vi "FRCts20_Backend_SetSglTeamData.vi"(8 "error in (no error)":errorcluster, 11 "Team":T1) -> (0 "error out":errorcluster, 2 "Status?":string)   [LabVIEW 2013, in "FRCts20_Backend_WebMethods.lvlib"]
doc: "The SetSglTeamData function applies a new team description to the data set, or overwrites existing team information with updated values. The function accepts a full team description as input, and provides a <b>Success!</b> or <b>Failed!</b> status return."
uses:
  FRCts20_Backend_WebMethods.lvlib
  FRCts20_Backend_FGVOperation.ctl
  FRCts20_Backend_Engine.lvlib
  FRCts20_Backend_IssueDfn.ctl
  FRCts20_Backend_Controls.lvlib
  FRCts20_Backend_TeamDfn.ctl
  FRCts20_Backend_Team_Info.ctl
  FRCts20_Backend_Note.ctl
  FRCts20_Backend_Note_list.ctl
  FRCts20_Backend_request_info.ctl
  FRCts20_Backend_IssueTeamList.ctl
panel:
  # "The SetSglTeamData function applies a new \nteam description to the data set, or overwrites \nexisting team information with updated values.\nThe function accepts a full team description as\ninput, and provides a Success! or Failed! status\nreturn."
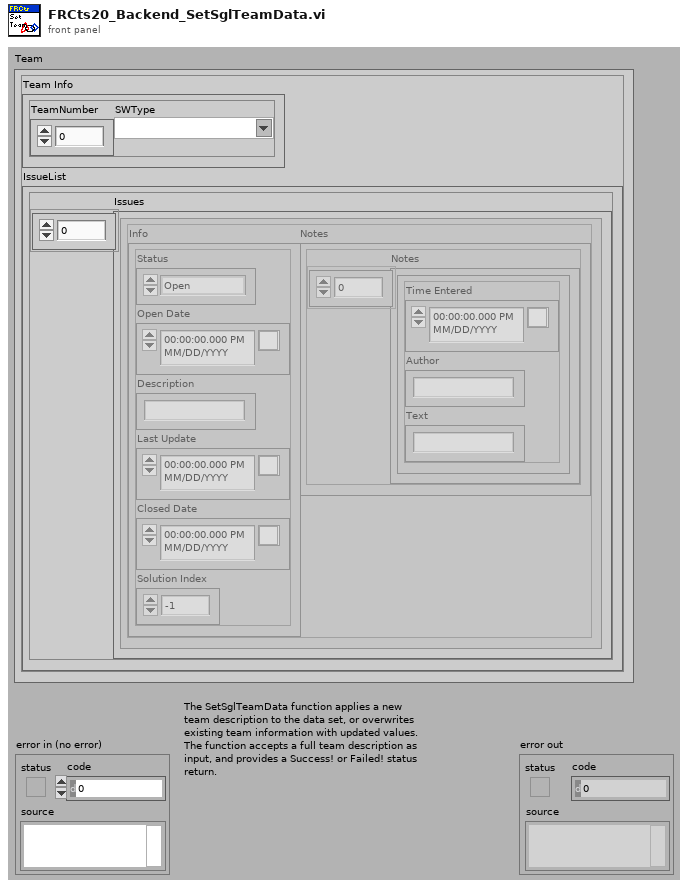
[diagram p1: front panel]
types:
  T1 = typedef "FRCts20_Backend_Controls.lvlib/FRCts20_Backend_TeamDfn.ctl" = cluster{"Team Info":T2, "IssueList":T3}
  T2 = typedef "FRCts20_Backend_Controls.lvlib/FRCts20_Backend_Team_Info.ctl" = cluster{"TeamNumber":u16, "SWType":string}
  T3 = typedef "FRCts20_Backend_Controls.lvlib/FRCts20_Backend_IssueTeamList.ctl" = cluster{"Issues":T4[]}
  T4 = typedef "FRCts20_Backend_Controls.lvlib/FRCts20_Backend_IssueDfn.ctl" = cluster{"Notes":T5, "Info":T7}
  T5 = typedef "FRCts20_Backend_Controls.lvlib/FRCts20_Backend_Note_list.ctl" = cluster{"Notes":T6[]}
  T6 = typedef "FRCts20_Backend_Controls.lvlib/FRCts20_Backend_Note.ctl" = cluster{"Time Entered":timestamp, "Author":string, "Text":string}
  T7 = typedef "FRCts20_Backend_Controls.lvlib/FRCts20_Backend_request_info.ctl" = cluster{"Status":enum16{"Open", "In Work", "Closed"}, "Open Date":timestamp, "Description":string, "Last Update":timestamp, "Closed Date":timestamp, "Solution Index":i32}
  T8 = typedef "FRCts20_Backend_Engine.lvlib/FRCts20_Backend_FGVOperation.ctl" = enum16{"Initialize", "EnqueueMessage", "EnqueueDataReturn", "FlushMessage", "FlushDataReturn"}
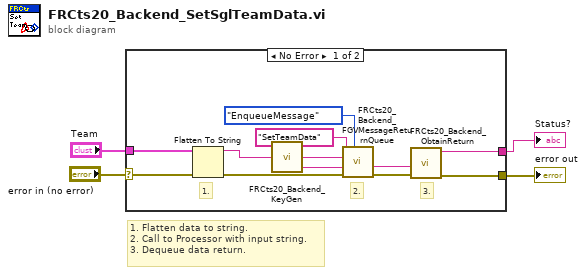
[diagram p0: block diagram]
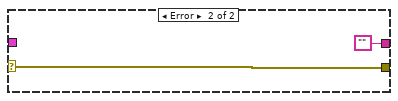
[diagram p2: hidden frame]
diagram:
  # "1. Flatten data to string.\n2. Call to Processor with input string.\n3. Dequeue data return."
  n1 = case shown="No Error" "error in (no error)" {
    selector: "error in (no error)" -> [w9 w17]
    tunnel: [w11 w17] -> w3
    tunnel: [w5 ""] -> w2
    tunnel: "Team" -> [w10 _]
    frame No Error {
      # "3."
      # "2."
      # "1."
      n2 = Flatten To String(anything=w10, error in (no error)=w9) -> (data string=w7:string, error out=w8:errorcluster)  [unwired: 2 in, 1 out]
      n3 = call "FRCts20_Backend_KeyGen.vi"() -> ("Keygen"=w13:string)  [unwired: 27 in]
      n4 = call "FRCts20_Backend_FGVMessageReturnQueue.vi"("Operation"=FRCts20_Backend_FGVOperation."EnqueueMessage", "error in (no error)"=w8, "Key"=w13, "Message Value"=w7, "Message Name"="SetTeamData") -> ("error out"=w12:errorcluster, "Key (Duplicate)"=w6:string)  [unwired: 3 in]
      n5 = call "FRCts20_Backend_ObtainReturn.vi"("error in (no error)"=w12, "Key"=w6) -> ("error out"=w11:errorcluster, "Message Value"=w5:string)  [unwired: 8 in]
    }
    frame Error {
    }
  }
  "error out" <- w3
  "Status?" <- w2
